vi "io.responseValidator.vi"(8 "error in":errorcluster, 10 "ResponsToValidate in":string, 11 "IoConf in 2":T1={"ADDR"=0, "Label"="Name", "Type"=enum."Type", "Mode"=enum."RIO", "Value"="Value", "Tags"="Tags", "calibration"=[]} {"calibration"."Y" format="%#.3f"; "calibration"."X" format="%#.3f"; "ADDR" format="%04d"}) -> (0 "error out":errorcluster, 2 "Data out":string)   [LabVIEW 2024]
uses:
  controls/IONode.ctl
  controls/type.address.ctl
  controls/enum.io.type.ctl
  controls/enum.io.mode.ctl
  controls/typeXyPoint.ctl
  controls/rio-rx-enum.ctl
panel:
  out "ResponseSize(minimumSize+dataSize)":u8
  out "DataSize":u8
  out "responseSize 2":u8
  out "DataSize 2":u8
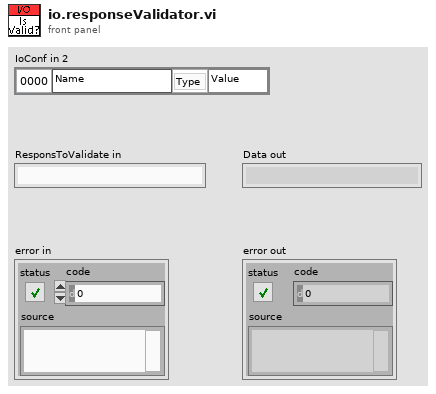
[diagram p1: front panel]
types:
  T1 = typedef "IONode.ctl" = cluster{"ADDR":T2, "Label":string, "Type":T3, "Mode":T4, "Value":string, "Tags":string, "calibration":T5[]}
  T2 = typedef "type.address.ctl" = u16
  T3 = typedef "enum.io.type.ctl" = enum16{"Type", "DI", "DO", "AI", "AO", "VL", "BUF"}
  T4 = typedef "enum.io.mode.ctl" = enum16{"Mode", "RIO", "SIM"}
  T5 = typedef "typeXyPoint.ctl" = cluster{"X":dbl, "Y":dbl}
  T6 = typedef "rio-rx-enum.ctl" = u16
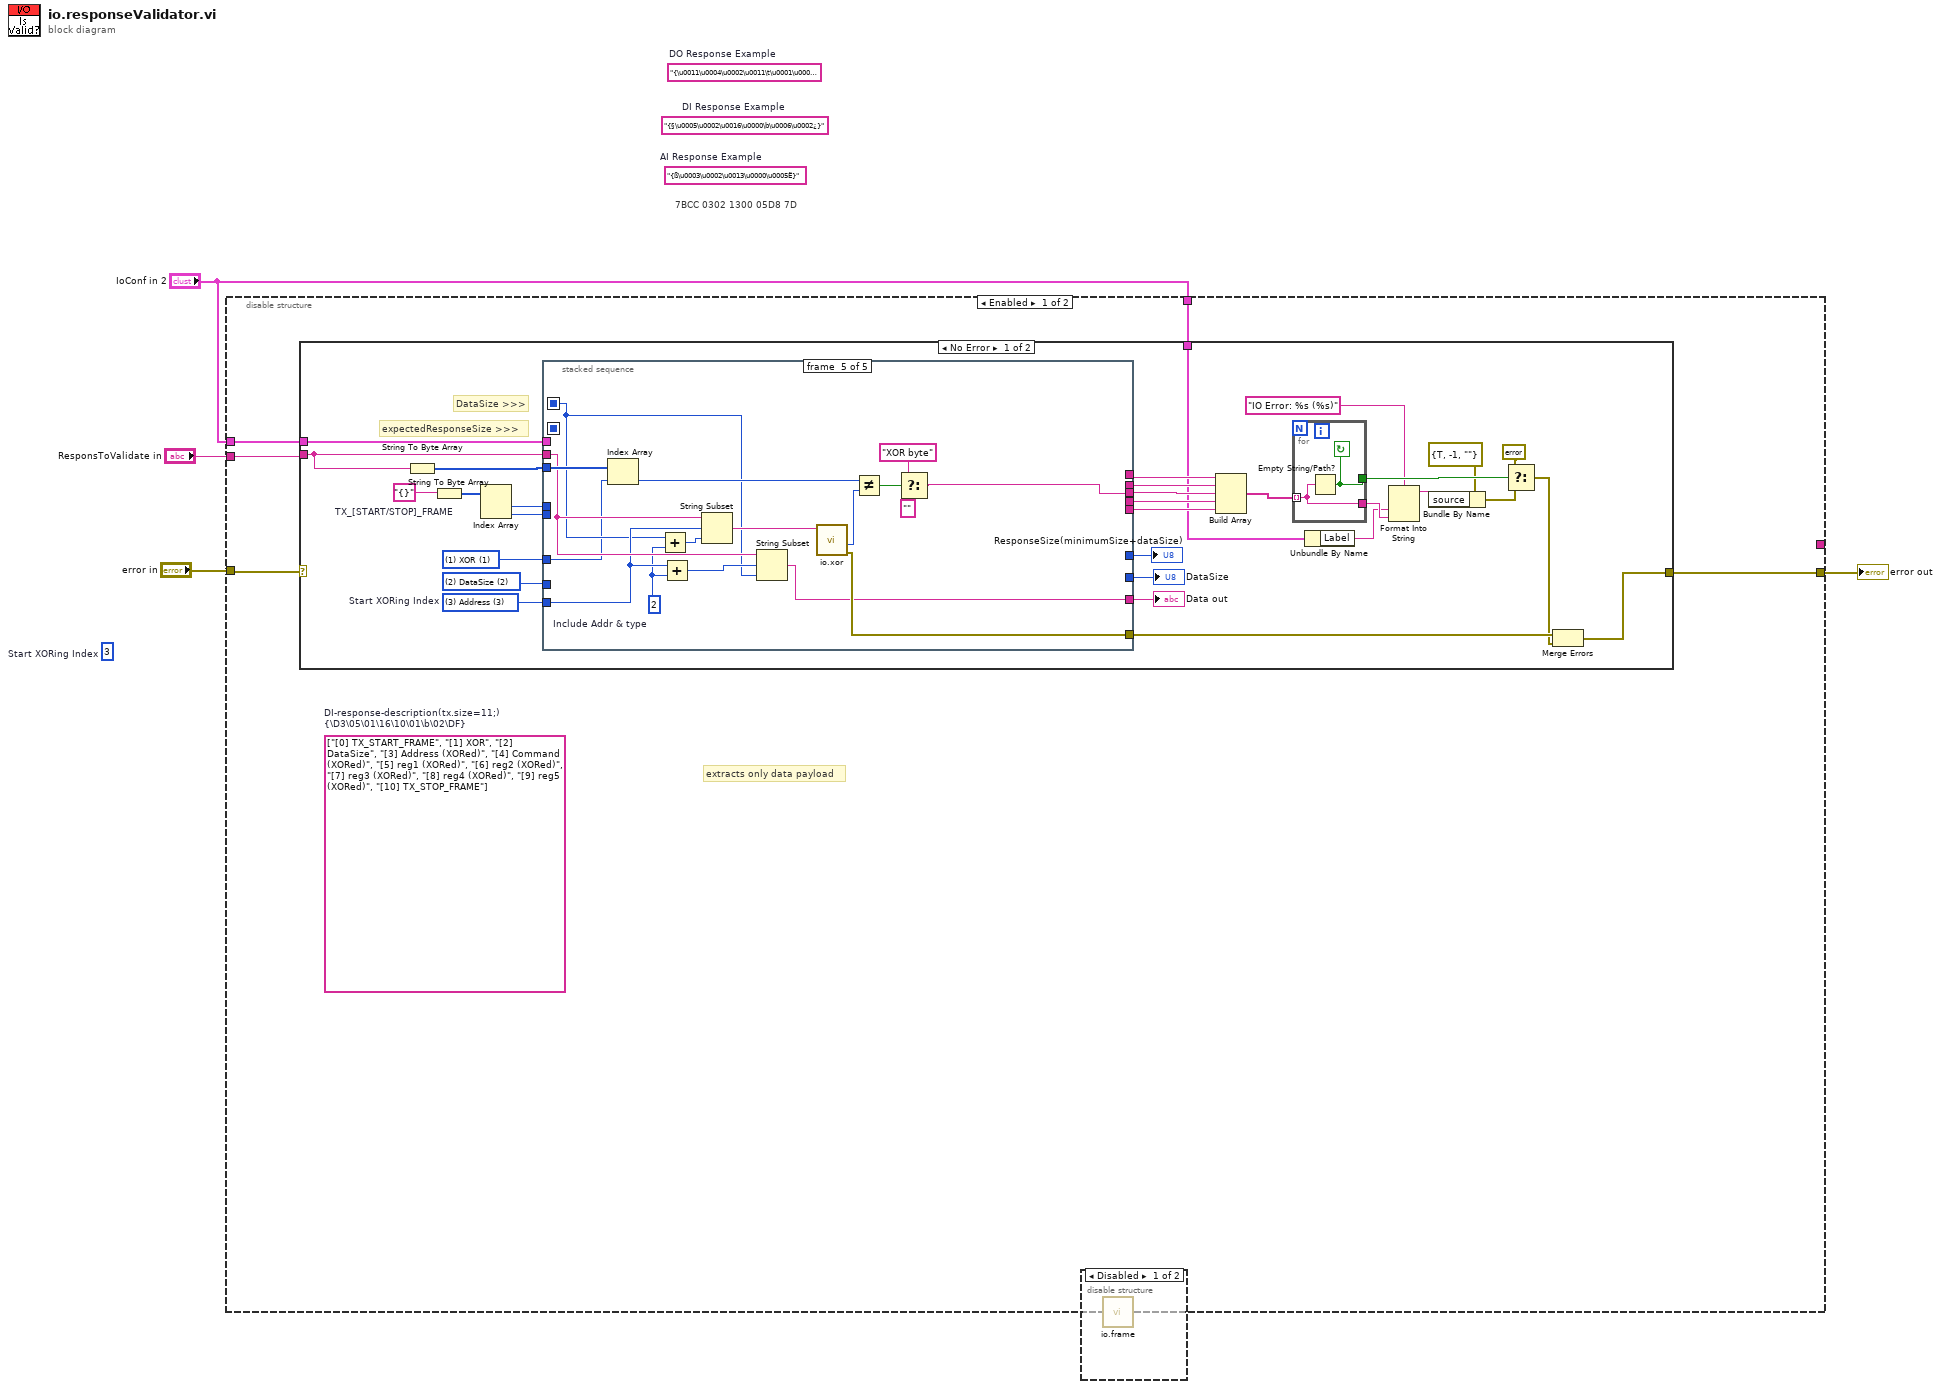
[diagram p0: block diagram]
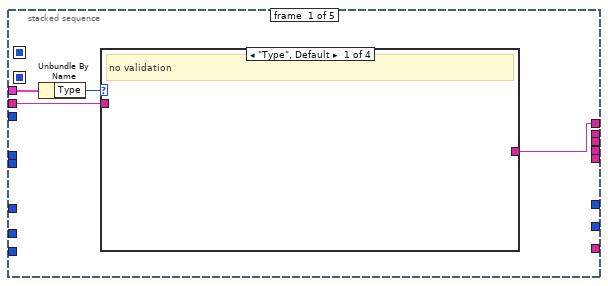
[diagram p2: hidden frame]
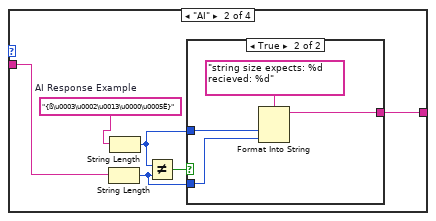
[diagram p3: hidden frame]
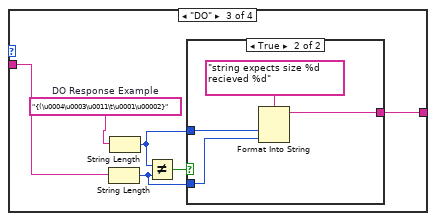
[diagram p5: hidden frame]
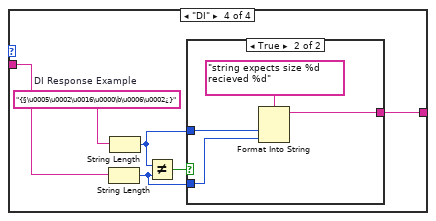
[diagram p7: hidden frame]
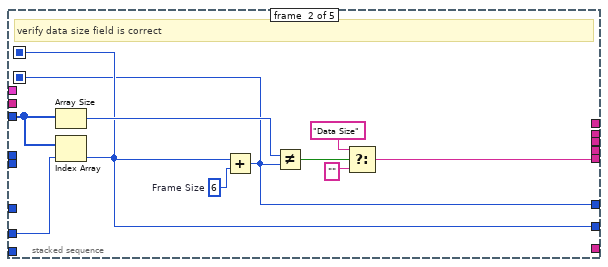
[diagram p9: hidden frame]
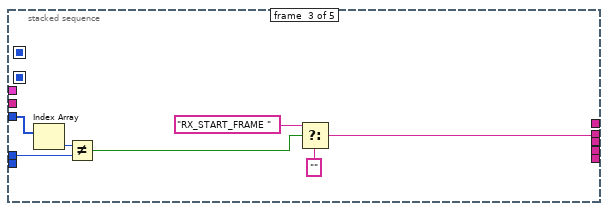
[diagram p10: hidden frame]
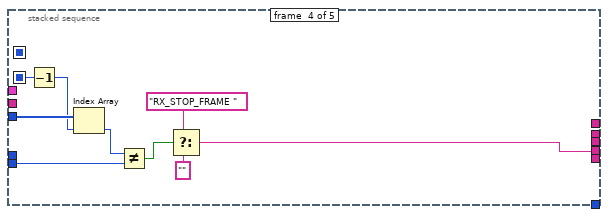
[diagram p11: hidden frame]
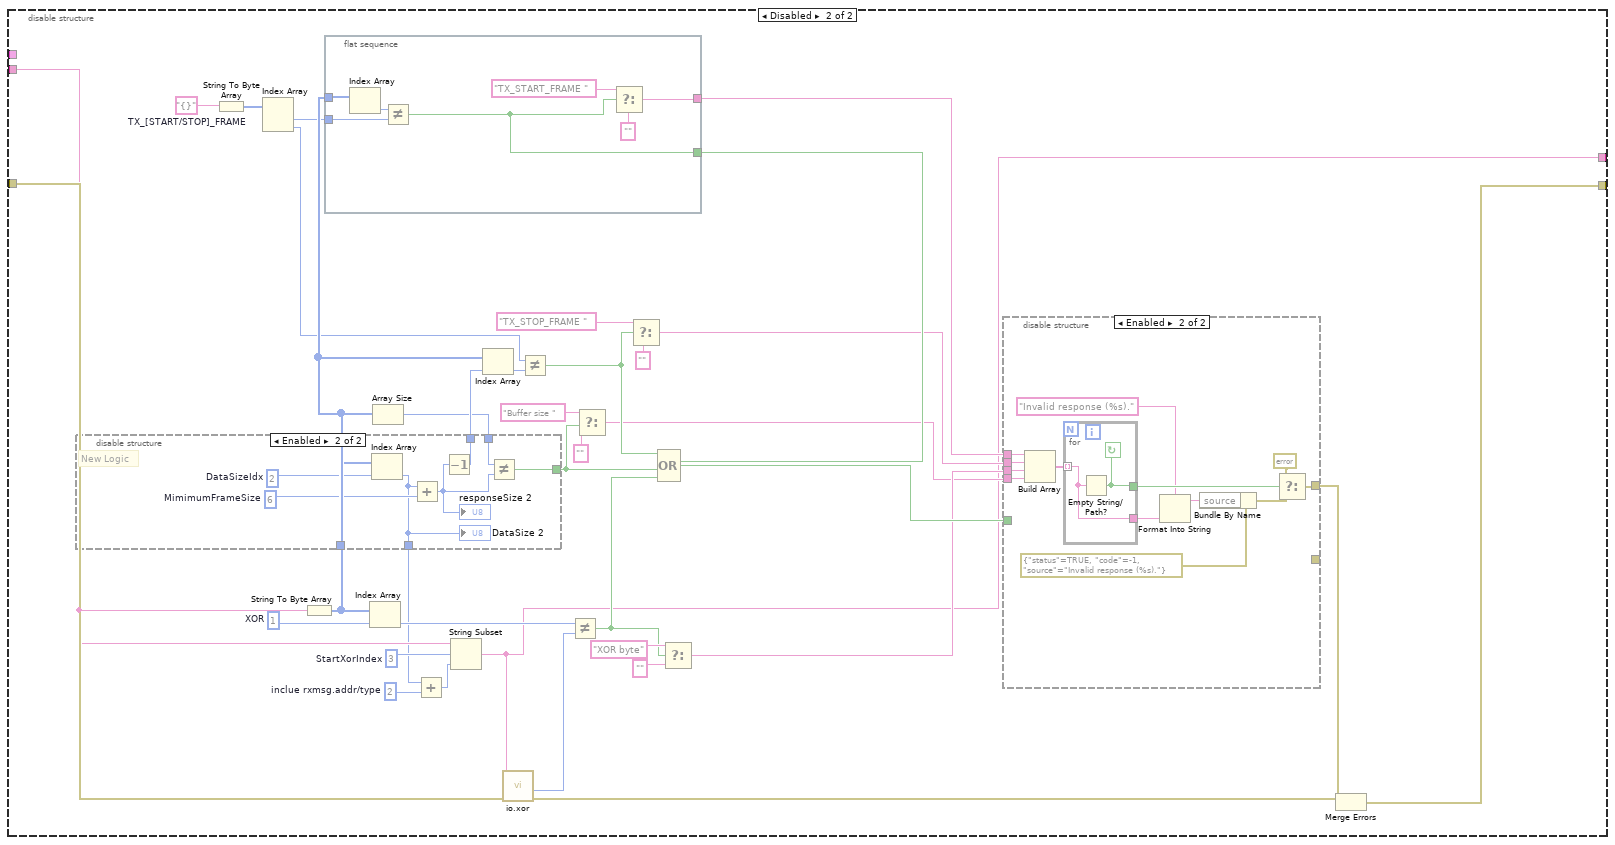
[diagram p13: hidden frame]
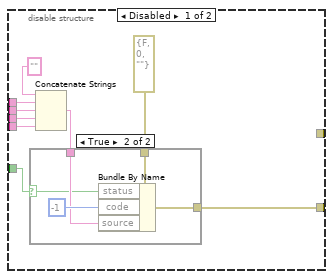
[diagram p14: hidden frame]
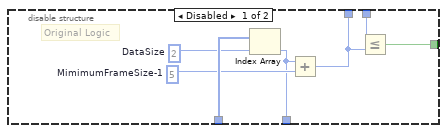
[diagram p16: hidden frame]
diagram:
  (unwired) "{ß\u0003\u0002\u0013\u0000\u0005Ë}"  # AI Response Example
  (unwired) "{§\u0005\u0002\u0016\u0000\b\u0006\u0002¿}"  # DI Response Example
  (unwired) "{\u0011\u0004\u0002\u0011\t\u0001\u0000\n}"  # DO Response Example
  (unwired) 3  # Start XORing Index
  # "7BCC 0302 1300 05D8 7D"
  n1 = disable-structure shown="Enabled" {
    disable-tunnel: "error in" -> [w7 w156]
    disable-tunnel: [w8 w155] -> w3
    disable-tunnel: "ResponsToValidate in" -> [w9 w135]
    disable-tunnel: [_ w121] -> _
    disable-tunnel: "IoConf in 2" -> [w6 _]
    disable-tunnel: "IoConf in 2" -> [w5 _]
    frame Enabled {
      (unwired) string[] ["[0] TX_START_FRAME", "[1] XOR", "[2]  DataSize", "[3] Address (XORed)", "[4] Command (XORed)", "[5] reg1 (XORed)", "[6] reg2 (XORed)", "[7] reg3 (XORed)", "[8] reg4 (XORed)", "[9] reg5 (XORed)", "[10] TX_STOP_FRAME"]  # DI-response-description(tx.size=11;) {\D3\05\01\16\10\01\b\02\DF}
      # "extracts only data payload"
      n2 = case shown="No Error" w7 {
        selector: w7 -> [_ w120]
        tunnel: w9 -> [w36 _]
        tunnel: [w20 w120] -> w8
        tunnel: w6 -> [w13 _]
        tunnel: w5 -> [w11 _]
        frame No Error {
          w14 = T6 3 items=["(0) RxStart", "(1) XOR", "(2) DataSize", "(3) Address", "(4) Type"]  # Start XORing Index
          w15 = T6 2 items=["(0) RxStart", "(1) XOR", "(2) DataSize", "(3) Address", "(4) Type"] ("Enum")
          w16 = T6 1 items=["(0) RxStart", "(1) XOR", "(2) DataSize", "(3) Address", "(4) Type"] ("Enum")
          w38 = "{}"  # TX_[START/STOP]_FRAME
          # "expectedResponseSize >>>"
          # "DataSize >>>"
          n3 = String To Byte Array(string=w36) -> (unsigned byte array=w40:u8[])
          n4 = String To Byte Array(string=w38) -> (unsigned byte array=w39:u8[])
          n5 = Index Array(array=w39) -> (element #1=w37:u8, element #2=w34:u8)  [unwired: 2 in]
          n6 = stacked-sequence {
            seq-local: [_ w78 _ _ _] -> [_ _ _ w99 _]
            seq-local: [_ w79 _ _ _] -> [_ _ _ _ w105]
            tunnel: w40 -> [_ w86 w93 w100 w119]
            tunnel: [_ _ w92 _ _] -> w32
            tunnel: w37 -> [_ _ w87 _ _]
            tunnel: [_ _ _ _ w110] -> w35
            tunnel: w36 -> [w43 _ _ _ w109]
            tunnel: [_ w82 _ _ _] -> w33
            tunnel: w34 -> [_ _ _ w96 _]
            tunnel: [_ _ _ w94 _] -> w31
            tunnel: [_ _ _ _ w112] -> w22
            tunnel: w15 -> [_ w80 _ _ _]
            tunnel: w14 -> [_ _ _ _ w108]
            tunnel: [_ w79 _ _ _] -> w19
            tunnel: [_ w78 _ _ _] -> w18
            tunnel: [_ _ _ _ w106] -> w17
            tunnel: w16 -> [_ _ _ _ w104]
            tunnel: w13 -> [w46 _ _ _ _]
            tunnel: [w44 _ _ _ _] -> w12
            frame #0 {
              n7 = Unbundle By Name(w46) -> ("Type"=w45:T3)
              n8 = case shown="\"Type\", Default" w45 {
                tunnel: [_ w49 w59 w70] -> w44
                tunnel: w43 -> [_ w48 w58 w69]
                frame "Type", Default {
                  # "no validation"
                }
                frame "AI" {
                  w50 = "{ß\u0003\u0002\u0013\u0000\u0005Ë}"  # AI Response Example
                  n9 = String Length(string=w48) -> (length=w47:i32)
                  n10 = String Length(string=w50) -> (length=w51:i32)
                  n11 = Not Equal?(x=w51, y=w47) -> (x != y?=w52:bool)
                  n12 = case shown="True" w52 {
                    tunnel: w51 -> [_ w55]
                    tunnel: [_ w54] -> w49
                    tunnel: w47 -> [_ w53]
                    frame False {
                    }
                    frame True {
                      n13 = Format Into String(format string="string size expects: %d recieved: %d" ("source"), w55, w53) -> (resulting string=w54:string)  [unwired: 2 in, 1 out]
                    }
                  }
                }
                frame "DO" {
                  w60 = "{(\u0004\u0003\u0011\t\u0001\u00002}"  # DO Response Example
                  n14 = String Length(string=w58) -> (length=w57:i32)
                  n15 = String Length(string=w60) -> (length=w61:i32)
                  n16 = Not Equal?(x=w61, y=w57) -> (x != y?=w62:bool)
                  n17 = case shown="True" w62 {
                    tunnel: w61 -> [_ w65]
                    tunnel: [_ w64] -> w59
                    tunnel: w57 -> [_ w63]
                    frame False {
                    }
                    frame True {
                      n18 = Format Into String(format string="string expects size %d recieved %d" ("source"), w65, w63) -> (resulting string=w64:string)  [unwired: 2 in, 1 out]
                    }
                  }
                }
                frame "DI" {
                  w67 = "{§\u0005\u0002\u0016\u0000\b\u0006\u0002¿}"  # DI Response Example
                  n19 = String Length(string=w69) -> (length=w68:i32)
                  n20 = String Length(string=w67) -> (length=w71:i32)
                  n21 = Not Equal?(x=w71, y=w68) -> (x != y?=w72:bool)
                  n22 = case shown="True" w72 {
                    tunnel: w71 -> [_ w75]
                    tunnel: [_ w74] -> w70
                    tunnel: w68 -> [_ w73]
                    frame False {
                    }
                    frame True {
                      n23 = Format Into String(format string="string expects size %d recieved %d" ("source"), w75, w73) -> (resulting string=w74:string)  [unwired: 2 in, 1 out]
                    }
                  }
                }
              }
            }
            frame #1 {
              w77 = u8 6  # Frame Size
              # "verify data size field is correct"
              n24 = Array Size(array=w86) -> (size(s)=w81:i32)
              n25 = Index Array(array=w86, index=w80) -> (element=w79:u8)
              n26 = Add(x=w79, y=w77) -> (x+y=w78:u8)
              n27 = Not Equal?(x=w81, y=w78) -> (x != y?=w83:bool)
              n28 = Select(t="Data Size" ("CMD"), s=w83, f="") -> (s? t:f=w82:string)
            }
            frame #2 {
              n29 = Index Array(array=w93) -> (element=w89:u8)  [unwired: 1 in]
              n30 = Not Equal?(x=w89, y=w87) -> (x != y?=w88:bool)
              n31 = Select(t="RX_START_FRAME " ("CMD"), s=w88, f="") -> (s? t:f=w92:string)
            }
            frame #3 {
              n32 = Decrement(x=w99) -> (x-1=w95:u8)
              n33 = Index Array(array=w100, index=w95) -> (element=w98:u8)
              n34 = Not Equal?(x=w98, y=w96) -> (x != y?=w97:bool)
              n35 = Select(t="RX_STOP_FRAME " ("CMD"), s=w97, f="") -> (s? t:f=w94:string)
            }
            frame #4 {
              w103 = u8 2  # Include Addr & type
              n36 = Index Array(array=w119, index=w104) -> (element=w114:u8)
              n37 = Add(x=w105, y=w103) -> (x+y=w118:u8)
              n38 = Add(x=w108, y=w103) -> (x+y=w107:T6)
              n39 = String Subset(string=w109, offset (0)=w108, length (rest)=w118) -> (substring=w111:string)
              n40 = String Subset(string=w109, offset (0)=w107, length (rest)=w105) -> (substring=w106:string)
              n41 = call "io.xor.vi"("payload in"=w111) -> ("error out"=w112:errorcluster, "Xor(payload) num"=w117:u8)  [unwired: 8 in, 1 out]
              n42 = Not Equal?(x=w114, y=w117) -> (x != y?=w113:bool)
              n43 = Select(t="XOR byte" ("CMD"), s=w113, f="") -> (s? t:f=w110:string)
            }
          }
          "DataSize" <- w19
          "ResponseSize(minimumSize+dataSize)" <- w18
          "Data out" <- w17
          n44 = Build Array(w12, w32, w35, w31, w33) -> (w23:string[])
          n45 = for {
            tunnel: w23 -> [w42] mode=indexing
            tunnel: [w42] -> w26
            tunnel: [w41] -> w30
            stop <- w41 continue-if-true
            n46 = Empty String/Path?(string/path=w42) -> (empty?=w41:bool)
          }
          n47 = Unbundle By Name(w11) -> ("Label"=w10:string)
          n48 = Format Into String(format string="IO Error: %s (%s)" ("source"), w10, w26) -> (resulting string=w24:string)  [unwired: 2 in, 1 out]
          n49 = Bundle By Name(cluster=errorcluster {"status"=TRUE, "code"=-1, "source"=""} ("error constant"), "source"=w24) -> (w27:errorcluster)
          n50 = Select(t=errorcluster {"status"=FALSE, "code"=0, "source"=""} ("error constant"), s=w30, f=w27) -> (s? t:f=w21:errorcluster)
          n51 = Merge Errors(w22, w21) -> (w20:errorcluster)
        }
        frame Error {
        }
      }
    }
    frame Disabled {
      w129 = "{}"  # TX_[START/STOP]_FRAME
      w141 = u8 2  # inclue rxmsg.addr/type
      w139 = 3  # StartXorIndex
      w136 = 1  # XOR
      n52 = String To Byte Array(string=w129) -> (unsigned byte array=w130:u8[])
      n53 = Index Array(array=w130) -> (element #1=w128:u8, element #2=w127:u8)  [unwired: 2 in]
      n54 = String To Byte Array(string=w135) -> (unsigned byte array=w153:u8[])
      n55 = flat-sequence {
        tunnel: w153 -> [w163]
        tunnel: [w162] -> w150
        tunnel: [w158] -> w133
        tunnel: w128 -> [w157]
        frame #0 {
          n56 = Index Array(array=w163) -> (element=w159:u8)  [unwired: 1 in]
          n57 = Not Equal?(x=w159, y=w157) -> (x != y?=w158:bool)
          n58 = Select(t="TX_START_FRAME " ("CMD"), s=w158, f="") -> (s? t:f=w162:string)
        }
      }
      n59 = Index Array(array=w153, index=w136) -> (element=w143:u8)
      n60 = Array Size(array=w153) -> (size(s)=w137:i32)
      n61 = disable-structure shown="Enabled" {
        disable-tunnel: w153 -> [w200 w208]
        disable-tunnel: [w199 w207] -> w146
        disable-tunnel: [w198 w202] -> w138
        disable-tunnel: w137 -> [w197 w205]
        disable-tunnel: [w194 w201] -> w131
        frame Disabled {
          w196 = 5  # MimimumFrameSize-1
          w195 = 2  # DataSize
          # "Original Logic"
          n62 = Index Array(array=w200, index=w195) -> (element=w194:u8)
          n63 = Add(x=w194, y=w196) -> (x+y=w198:i32)
          n64 = Less Or Equal?(x=w197, y=w198) -> (x <= y?=w199:bool)
        }
        frame Enabled {
          w204 = u8 6  # MimimumFrameSize
          w203 = 2  # DataSizeIdx
          # "New Logic"
          n65 = Index Array(array=w208, index=w203) -> (element=w201:u8)
          "DataSize 2" <- w201
          n66 = Add(x=w201, y=w204) -> (x+y=w206:u8)
          "responseSize 2" <- w206
          n67 = Decrement(x=w206) -> (x-1=w202:u8)
          n68 = Not Equal?(x=w205, y=w206) -> (x != y?=w207:bool)
        }
      }
      n69 = Add(x=w131, y=w141) -> (x+y=w140:u8)
      n70 = String Subset(string=w135, offset (0)=w139, length (rest)=w140) -> (substring=w121:string)
      n71 = Index Array(array=w153, index=w138) -> (element=w126:u8)
      n72 = call "io.xor.vi"("error in"=w156, "payload in"=w121) -> ("error out"=w134:errorcluster, "Xor(payload) num"=w142:u8)  [unwired: 7 in, 1 out]
      n73 = Not Equal?(x=w127, y=w126) -> (x != y?=w132:bool)
      n74 = Not Equal?(x=w143, y=w142) -> (x != y?=w149:bool)
      n75 = Select(t="Buffer size " ("CMD"), s=w146, f="") -> (s? t:f=w122:string)
      n76 = Select(t="TX_STOP_FRAME " ("CMD"), s=w132, f="") -> (s? t:f=w125:string)
      n77 = Compound Arithmetic op=OR(w132, w133, w146, w149) -> (w154:bool)
      n78 = Select(t="XOR byte" ("CMD"), s=w149, f="") -> (s? t:f=w123:string)
      n79 = disable-structure shown="Enabled" {
        disable-tunnel: [w172 _] -> _
        disable-tunnel: w154 -> [w171 _]
        disable-tunnel: w122 -> [w168 w188]
        disable-tunnel: w150 -> [w167 w191]
        disable-tunnel: w125 -> [w165 w190]
        disable-tunnel: w123 -> [w164 w189]
        disable-tunnel: [_ w184] -> w124
        frame Disabled {
          n80 = Concatenate Strings("" ("string"), w167, w165, w164, w168) -> (w169:string)
          n81 = case shown="True" w171 {
            selector: w171 -> [_ w174]
            tunnel: [w173 w178] -> w172
            tunnel: w169 -> [_ w176]
            tunnel: errorcluster {"status"=FALSE, "code"=0, "source"=""} ("error constant") -> [w173 w175]
            frame False {
            }
            frame True {
              n82 = Bundle By Name(cluster=w175, "status"=w174, "code"=-1, "source"=w176) -> (w178:errorcluster)
            }
          }
        }
        frame Enabled {
          n83 = Build Array(w191, w190, w189, w188) -> (w187:string[])
          n84 = for {
            tunnel: w187 -> [w193] mode=indexing
            tunnel: [w193] -> w181
            tunnel: [w192] -> w186
            stop <- w192 continue-if-true
            n85 = Empty String/Path?(string/path=w193) -> (empty?=w192:bool)
          }
          n86 = Format Into String(format string="Invalid response (%s)." ("source"), w181) -> (resulting string=w179:string)  [unwired: 2 in, 1 out]
          n87 = Bundle By Name(cluster=errorcluster {"status"=TRUE, "code"=-1, "source"="Invalid response (%s)."} ("error constant"), "source"=w179) -> (w182:errorcluster)
          n88 = Select(t=errorcluster {"status"=FALSE, "code"=0, "source"=""} ("error constant"), s=w186, f=w182) -> (s? t:f=w184:errorcluster)
        }
      }
      n89 = Merge Errors(w134, w124) -> (w155:errorcluster)
    }
  }
  "error out" <- w3
  n90 = disable-structure shown="Disabled" {
    frame Disabled {
      n91 = call "io.frame.vi"() -> ()  [unwired: 10 in, 2 out]
    }
    frame Enabled {
    }
  }
